vi "On Drop.vi"(8 "error in (no error)":errorcluster, 10 "Actor in":refnum<class "Actor.lvclass">, 11 "WebSocket Connection Handler Msg in":refnum<class "WebSocket Connection Handler Msg.lvclass">) -> (0 "error out":errorcluster, 2 "Actor out":refnum<class "Actor.lvclass">, 3 "WebSocket Connection Handler Msg out":refnum<class "WebSocket Connection Handler Msg.lvclass">)   [LabVIEW 2016, in "WebSocket Actors.lvlib" / "WebSocket Connection Handler Msg.lvclass"]
uses:
  WebSocket Connection Handler Msg.lvclass
  <vilib>/ActorFramework/Actor/Actor.lvclass
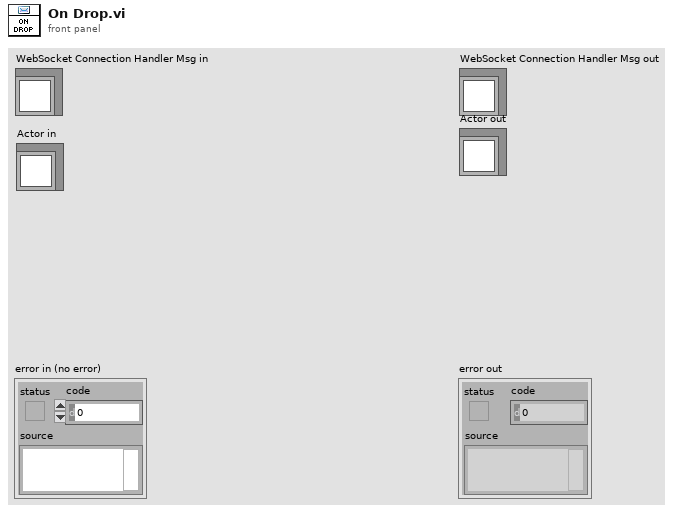
[diagram p1: front panel]
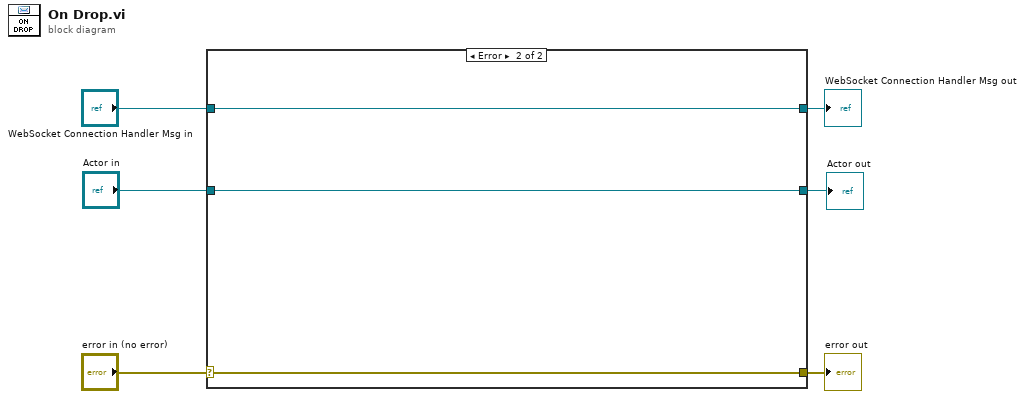
[diagram p0: block diagram]
diagram:
  n1 = case shown="Error" "error in (no error)" {
    selector: "error in (no error)" -> [w8 w12]
    tunnel: [w8 w12] -> w5
    tunnel: [w9 w11] -> w3
    tunnel: "WebSocket Connection Handler Msg in" -> [w9 w11]
    tunnel: "Actor in" -> [w7 w10]
    tunnel: [w7 w10] -> w1
    frame No Error {
      # "Wire the error cluster across even in the \"No Error\"\ncase so that warnings get propagated."
    }
    frame Error {
    }
  }
  "error out" <- w5
  "WebSocket Connection Handler Msg out" <- w3
  "Actor out" <- w1
